vi "Uint8Array Create (Dimensions).vi"(8 "error in (no error)":errorcluster, 10 "Array dimensions":i32[](array[numeric]), 11 "U8 array in":u8[](array[numeric])) -> (0 "error out":errorcluster, 3 "Uint8Array DVR out":refnum<data-value>)   [LabVIEW 2010, in "MDSplus.lvlib"]
uses:
  <vilib>/MDSplus/Library/MDSplus.lvlib
  <vilib>/MDSplus/Classes/Data_Class/Array_Class/Uint8Array_Class/Uint8Array.lvclass
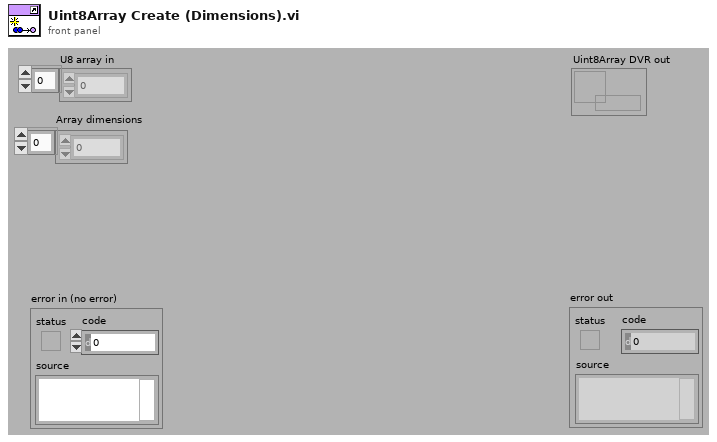
[diagram p1: front panel]
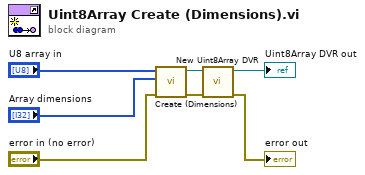
[diagram p0: block diagram]
diagram:
  n1 = call <vilib>:"Create (Dimensions).vi"("error in (no error)"="error in (no error)", "Dimensions"="Array dimensions", "U8 array in"="U8 array in") -> ("error out"=w4:errorcluster, "Uint8Array out"=w5:refnum<class "Uint8Array.lvclass">)  [unwired: 7 in]
  n2 = call <vilib>:"New Uint8Array DVR.vi"("error in (no error)"=w4, "Uint8Array in"=w5) -> ("error out"=→"error out":errorcluster, "Uint8Array DVR out"=→"Uint8Array DVR out":refnum<data-value>)  [unwired: 8 in]
